vi "Day 2 - part b solution.vi"() -> ()   [LabVIEW 2020]
panel:
  in  "Input":string="A Y\nB X\nB X\nC Y\nB X\nA Z\nB X\nB X\nC Z\nA Z\nC Z\nA X\nA Y\nA Y\nB X\nC Y\nB Z\nA X\nB X\nC Y\nC Y\nA Y\nA Y\nC Y\nB X\nB X\nB X\nA X\nB X\nB X\nC Y\nC Y\nB X\nA Z\nA Z\nB X\nA Z\nC Y\nB X\nB X\nB X\nB X\nB X\nB Z\nA Z\nB X\nA Z\nA X\nB X\nA Z\nB X\nC Y\nA Z\nA Z\nB X\nB X\nB Z\nC Y\nA Y\nB Z\nA Z\nC Z\nB X\nC Y\nC Y\nB Z\nB X\nB X\nB Z\nB X\nB X\nA Y\nA Z\nB Z\nB X\nB Y\nB Z\nB X\nC X\nB Z\nB X\nA Z\nB Z\nB Z\nB X\nA Y\nA Z\nA Y\nB X\nB Z\nB X\nB X\nA Y\nA Y\nB X\nB X\nB X\nC X\nC Y\nB X\nB X\nB Z\nB X\nB X\nB X\nC Y\nB X\nC Y\nA Z\nB X\nB Z\nB X\nC Y\nC Y\nA Z\nA Y\nC Y\nB X\nB X\nB Z\nA Y\nB X\nB X\nB X\nA Y\nB Z\nB X\nA Y\nB Z\nC Y\nA X\nB X\nB X\nA Z\nC Y\nB X\nB Z\nA Y\nA Y\nC Y\nA Y\nC Y\nB X\nB Z\nB X\nC Y\nA Y\nB X\nC Z\nA Z\nC Y\nB X\nB Z\nB X\nB X\nB Z\nB Y\nA Y\nB X\nA Y\nA Z\nA Z\nB X\nC Y\nB Z\nA X\nA Y\nB X\nA Z\nB X\nA Y\nB Y\nB X\nA Y\nB X\nB X\nB X\nB X\nB X\nB X\nB X\nA Z\nB X\nB X\nB Z\nB Z\nB Z\nB Z\nA Y\nB Z\nC Z\nB X\nB X\nB X\nA Z\nB Z\nC Y\nB X\nC Y\nB Z\nB X\nB Z\nB X\nC Z\nA Z\nA Y\nA X\nB X\nB Z\nA Y\nB X\nB X\nB X\nB X\nC Y\nC Y\nA Z\nA Y\nA X\nB X\nB X\nA Y\nB X\nC Y\nA X\nB X\nB X\nB X\nA Z\nC Y\nB Z\nC Y\nA Y\nC Y\nA X\nA Z\nC Z\nA Z\nB X\nB Z\nB X\nB X\nA X\nB X\nB X\nB Z\nA Y\nC Y\nA Z\nC Z\nA Z\nA Z\nA Z\nB Z\nB Z\nB Z\nC Z\nB Y\nC Y\nC Y\nC X\nB X\nC Y\nB X\nB X\nC Y\nB Z\nB X\nC Z\nB X\nA Z\nB Z\nC X\nC Y\nB X\nA Y\nA Z\nB X\nA Z\nA Z\nB X\nB X\nC Z\nB Z\nA Z\nA Z\nC Z\nB X\nA Z\nA X\nB X\nB X\nC Y\nB X\nB Z\nA Z\nB X\nB X\nB X\nB X\nB X\nB X\nB X\nB X\nC Y\nC Y\nB X\nB X\nB X\nC Y\nA X\nB Z\nB X\nB X\nC Z\nB X\nB Z\nB Z\nA Z\nB X\nB Z\nB X\nA Z\nB X\nB X\nB X\nB X\nB X\nC Z\nB X\nB X\nB X\nB Z\nC Y\nC Y\nA Y\nB X\nB Z\nC Y\nB X\nB X\nC Y\nC Y\nB X\nB X\nB X\nB X\nC X\nB Z\nB X\nB Z\nC Y\nA X\nA Z\nB X\nB X\nA Z\nB X\nC Z\nB X\nA Y\nA Z\nB X\nB X\nB X\nB Z\nB X\nA Y\nC Y\nB Z\nB Z\nC Y\nB X\nA Y\nC Y\nB X\nC Z\nB X\nB X\nA Z\nB Z\nB Z\nB X\nA Z\nA Z\nA Y\nB Z\nB X\nB X\nB X\nB X\nB Z\nB X\nB Z\nB X\nA Z\nB X\nB X\nC Z\nC Z\nB X\nC Y\nA Z\nB X\nB Z\nC Z\nC X\nB X\nA Y\nA Y\nB X\nB X\nC Y\nA X\nC Y\nA Y\nA Z\nC Z\nB Z\nA Z\nB X\nB X\nB Z\nC Y\nA Y\nA Y\nB Z\nA Z\nA Z\nB Z\nA Z\nB X\nA Y\nA Y\nC Y\nB X\nB X\nA X\nB X\nC X\nA Y\nA Z\nB X\nB X\nB X\nB X\nB X\nB Z\nB Z\nB Z\nB X\nB X\nA Z\nB X\nC Z\nA Z\nC Y\nB Z\nC Y\nA Y\nC Y\nB X\nB X\nB X\nA Y\nB Z\nB Z\nB X\nB Z\nB X\nB X\nB X\nC Y\nB X\nB Z\nA Z\nB X\nB X\nB X\nC Z\nC Z\nB Z\nB X\nA Z\nA X\nB X\nB X\nB Y\nA Y\nB X\nB X\nC Z\nA Z\nB X\nB Z\nB Z\nA Y\nA Z\nB Z\nB Z\nA Y\nA Y\nA Z\nC Y\nC Y\nB X\nB X\nA Z\nB X\nC Y\nC X\nA Z\nB X\nB X\nB X\nA Y\nC Y\nB Y\nC Y\nC X\nA X\nA Y\nB Z\nB X\nB Z\nA X\nB X\nC Z\nB X\nB X\nA Y\nB Z\nB X\nA Y\nA Y\nB X\nC Y\nB X\nB X\nC Y\nB X\nC Z\nB Z\nB X\nA X\nC Y\nC Y\nB X\nB Z\nB X\nB X\nA Z\nB X\nA Z\nB Z\nB X\nB X\nB Z\nA Y\nC Y\nB Z\nB X\nA Y\nB X\nA X\nC Z\nB X\nB Z\nB Z\nA X\nC Y\nA Z\nB X\nB Z\nA Y\nB X\nC Y\nA Y\nB Z\nC Y\nB X\nB X\nB X\nB X\nB X\nB X\nC Y\nB X\nC Z\nA Y\nC Y\nB X\nC Y\nB Z\nB X\nA X\nB Z\nB X\nC X\nB X\nA Z\nB X\nA Y\nB X\nC Z\nB X\nB Z\nA Y\nB X\nA Z\nA Z\nA Z\nA Y\nA Y\nB X\nA Z\nB X\nB X\nA Y\nA Y\nA Y\nB Z\nC Y\nB Z\nB X\nC Z\nA Y\nC Y\nB X\nB X\nB Z\nB X\nB X\nB X\nC Y\nC Y\nA Y\nB Z\nB Z\nB X\nB X\nB Z\nB X\nA Y\nC Y\nB X\nC X\nB Z\nB X\nB Z\nB Z\nC Y\nB Z\nB X\nC X\nB X\nC Y\nB X\nA Z\nB X\nB X\nB X\nB X\nB X\nC Y\nA Y\nB X\nC Y\nB Z\nB Z\nB X\nC X\nB Z\nC Y\nC X\nC Y\nA Z\nB Z\nC Y\nC X\nB X\nA Y\nC Y\nB X\nC Z\nB Z\nA Y\nC Z\nC X\nB X\nB X\nA Y\nC X\nB X\nB X\nA X\nA Z\nA X\nA Y\nA Y\nC Y\nB X\nC Z\nB X\nC Y\nA Y\nB X\nB X\nB X\nB X\nA Z\nC X\nB X\nB Z\nB X\nB X\nC Y\nB X\nC Z\nB X\nB X\nB X\nB X\nB X\nC Y\nB X\nB X\nA Y\nB X\nC Y\nC Y\nA Y\nB X\nA X\nA Y\nB X\nB Z\nB X\nB Z\nA X\nA Y\nA X\nB X\nC Z\nA Y\nB Z\nA Y\nB Z\nB Z\nB X\nB Z\nB X\nB X\nB X\nB Z\nB X\nB X\nB X\nA Z\nC Z\nC Z\nA X\nA X\nB X\nB X\nA X\nB X\nA X\nA Z\nB Z\nB X\nC Y\nB X\nC Y\nA Y\nC X\nA X\nA Y\nB Z\nB X\nB X\nC Z\nB Y\nA Y\nB Y\nC Y\nA Y\nB X\nB X\nC X\nB Z\nA Y\nB Z\nA Z\nB X\nB X\nA Z\nC Z\nA Y\nB X\nB X\nB Z\nB X\nB X\nB Z\nA X\nA Z\nC Y\nA Y\nA Z\nB X\nC Y\nB Z\nC Y\nB X\nB X\nB Z\nB X\nA Y\nB X\nA Y\nB X\nA Y\nB X\nA Y\nC Y\nA Y\nB Z\nA Y\nB X\nA Z\nC Y\nB X\nB X\nB X\nA X\nB X\nB Z\nA Z\nA Z\nB X\nB Z\nB X\nA Y\nB Z\nB X\nB X\nA Y\nA Y\nC Z\nC Y\nB X\nA X\nA Y\nA X\nC Y\nB X\nC X\nB X\nB X\nA Y\nA Y\nA Y\nB Y\nB X\nB X\nB X\nC Z\nB Z\nC Z\nA X\nB X\nB X\nA Y\nA Z\nB X\nA Y\nB Z\nB Z\nC Y\nB X\nB X\nC X\nB X\nC X\nB X\nB Z\nA X\nB X\nA Z\nA X\nB Z\nA Y\nB X\nB X\nB X\nB X\nB Z\nA Z\nB X\nB Z\nB X\nB Z\nC Y\nB X\nC Y\nB X\nB X\nB X\nA Y\nB X\nA Y\nB X\nB X\nA X\nC Z\nC Y\nA Z\nB X\nA Y\nC Z\nC Y\nC Y\nB Z\nA Y\nB X\nA Y\nB X\nB X\nB Z\nB Z\nB X\nC X\nB Z\nA X\nA Y\nA Y\nB Z\nA Z\nC Y\nB X\nB Z\nA Y\nC Y\nA Y\nA X\nA Z\nB X\nB X\nC Y\nB X\nC Y\nB X\nA X\nB Z\nC X\nB Y\nA Y\nC Y\nB X\nA X\nB X\nB X\nB X\nA Z\nA Y\nB X\nC Z\nB X\nC X\nC Z\nB X\nB X\nC Y\nB X\nB Z\nA Y\nA Y\nB X\nB X\nB Z\nC Y\nB X\nB X\nB X\nA Y\nC Y\nB X\nA Y\nA Z\nC Y\nB X\nA Y\nA Z\nB Z\nA Z\nB X\nC X\nB Z\nA Y\nB Z\nA Y\nC Y\nA X\nA Y\nB X\nC Y\nC Y\nB X\nA X\nB Z\nB X\nB X\nA Z\nA Z\nA Y\nA Y\nB X\nB X\nB X\nA X\nB X\nB X\nB X\nA X\nB Z\nC Z\nA Y\nC Y\nC Y\nC X\nB X\nB Z\nB Z\nB X\nB X\nC Y\nA X\nC Y\nA X\nB X\nB X\nB Z\nB Z\nC Y\nC Y\nA Z\nC Y\nA Z\nB X\nA Z\nA Y\nB Z\nB Z\nB X\nB X\nA Y\nB Z\nB X\nC Z\nA Z\nB Z\nB X\nB Z\nB X\nC Y\nB X\nA Y\nB Z\nC Y\nB Z\nC Z\nB X\nC Z\nB X\nB X\nB X\nC Y\nB X\nB X\nB Z\nA Y\nB X\nB Z\nA Z\nB X\nC Y\nC X\nC Y\nA Z\nB X\nA Z\nB X\nC Z\nA Y\nB Z\nB Z\nA Y\nC Z\nC X\nA Y\nB X\nB Z\nB X\nB X\nB X\nB X\nA X\nB X\nB X\nA Z\nB X\nB X\nA Z\nC Y\nA X\nB Z\nB X\nB X\nA Z\nB X\nA Y\nB Z\nC Y\nB X\nA Y\nC Y\nB Z\nB X\nA Z\nA Z\nB X\nB X\nB Z\nB X\nB X\nA Z\nB X\nB Z\nB Z\nC Y\nA Z\nB X\nA Y\nB X\nB X\nB X\nB Z\nA X\nC Y\nB Z\nB X\nB X\nB X\nB X\nB X\nB Z\nB X\nB Z\nA Z\nB Z\nB X\nC Z\nB Z\nC Z\nA Z\nC X\nA Y\nB Z\nB Z\nB X\nB Z\nB Z\nA Z\nC Z\nA X\nC Y\nC Y\nA Y\nA X\nA Z\nB X\nA Y\nB X\nB X\nC Y\nC Y\nB X\nB Z\nA Y\nB X\nB Z\nB X\nB X\nA Z\nC Y\nB X\nC Y\nA Y\nB Z\nA Z\nA Y\nB X\nA Z\nB Z\nB X\nA Y\nA Y\nA Z\nA X\nB Z\nC Z\nB X\nC Z\nB X\nB Z\nA X\nB X\nB X\nB X\nB X\nC Y\nB X\nA X\nB Z\nA Y\nB X\nA Z\nB X\nB Z\nA Y\nA Y\nA Y\nA Y\nA Z\nC Y\nC Z\nB X\nB Z\nA Y\nB X\nB X\nB X\nA Y\nB Z\nB X\nB Z\nB X\nB X\nB X\nC Y\nC Y\nC X\nB X\nA Y\nA Y\nC Z\nA Y\nA Y\nC X\nA Z\nB X\nB X\nB X\nB X\nC Y\nA Y\nB Z\nA Z\nB X\nC X\nA Z\nB X\nC Y\nB X\nB X\nC Y\nB X\nB X\nB X\nA Y\nB X\nB X\nC Z\nB X\nC Y\nC Y\nB X\nA Z\nB X\nB X\nC Y\nA Y\nB X\nB Z\nB X\nB X\nB X\nC Y\nC Z\nB Z\nC Y\nB X\nB Z\nB X\nB X\nB X\nC Y\nC X\nB X\nA Y\nA Z\nB Z\nA Y\nB X\nB X\nB Y\nC Y\nC X\nB Z\nA Z\nB X\nB X\nA Y\nC Z\nC Y\nB X\nC Y\nA Z\nA Y\nB Z\nB X\nB X\nB X\nB X\nA Z\nA X\nA X\nA X\nC Y\nB Z\nB X\nC Y\nB X\nB X\nA Z\nC Z\nC Z\nB X\nA Y\nB X\nB Z\nB X\nA Y\nA Y\nA Z\nC Y\nA Y\nA Z\nA Y\nA Y\nB X\nA Y\nB X\nA Z\nA Z\nC Y\nB X\nB X\nC Y\nB X\nB X\nB X\nC Y\nA Y\nB X\nA Y\nB Z\nC Y\nB X\nA Y\nB Z\nA Z\nB Z\nA Z\nB X\nC Y\nB X\nB X\nB X\nC Y\nA Y\nB X\nA Y\nC X\nA Z\nB X\nB Y\nB X\nB X\nA Z\nB X\nB X\nB Z\nB X\nC Y\nB X\nB X\nB Z\nB X\nC Y\nB X\nC Y\nB X\nB Z\nA Y\nB X\nB X\nC Z\nB X\nC Y\nA Y\nC Y\nB X\nB Z\nB X\nB X\nB X\nB X\nA Y\nB X\nA Z\nA Y\nA X\nC Y\nB X\nC Y\nB X\nA Z\nC Y\nC Y\nB Z\nB X\nA Y\nB Z\nA Y\nA Y\nB Z\nB Z\nB X\nC Y\nC Y\nB X\nA X\nA Z\nB X\nC Y\nB X\nB X\nB Z\nB X\nB Z\nC Y\nC Z\nC Y\nA Y\nA Z\nB X\nC Y\nA Y\nC X\nB X\nB X\nA Y\nB X\nB X\nB X\nB Z\nB Y\nA X\nA Y\nC Y\nC Y\nA Y\nC Y\nB Z\nB Z\nC Y\nB X\nC Y\nC Z\nA Y\nC X\nA Y\nA Y\nC Y\nC Y\nB X\nA Y\nA X\nB X\nB X\nB Z\nB X\nA Z\nA Y\nA Y\nB X\nB X\nB Z\nB Z\nB X\nB Z\nA Z\nA Y\nA Z\nB X\nC Y\nB Z\nB X\nA Y\nB X\nC X\nB X\nB X\nC Y\nB X\nB X\nB X\nA Y\nA X\nA Y\nB X\nB X\nA Y\nA Y\nA Z\nA Z\nC X\nC Y\nA Z\nC Y\nB Z\nB X\nA Y\nB X\nB Z\nC Z\nA Y\nA Z\nA Y\nB X\nB Z\nB X\nA X\nB Z\nB X\nC Y\nB X\nA Z\nC Z\nA X\nB X\nB X\nA Y\nC Y\nB X\nB X\nB X\nB X\nB X\nA X\nB X\nA Z\nC Z\nB Z\nB X\nC X\nA X\nC Y\nA Y\nA Z\nB X\nA X\nA Z\nA Z\nB X\nB X\nA Z\nC Y\nA Z\nB X\nC Y\nB X\nC Z\nC Y\nC X\nA Z\nC X\nB Z\nB X\nB X\nC Y\nB X\nC Y\nA Z\nA Z\nA Z\nA Y\nA Z\nB X\nB X\nB X\nB Z\nC Y\nC Z\nC Y\nC Y\nC Y\nA Y\nB Z\nA X\nB X\nB X\nB X\nA X\nA Y\nB X\nB Z\nA Z\nA Y\nA Y\nB Z\nB X\nB X\nC Y\nC Y\nC Y\nB X\nC Y\nB X\nB X\nB X\nC Y\nA Y\nA Y\nC Z\nC Y\nB X\nA X\nA Y\nB X\nC Y\nB X\nA Y\nC Y\nA Y\nB X\nB X\nB Z\nA Y\nB Z\nB Z\nB X\nB X\nC X\nC Y\nB X\nB X\nA X\nC Y\nB X\nB Z\nB X\nB X\nA Y\nB X\nB Z\nB Z\nC Y\nB X\nB Z\nB Z\nB Z\nB X\nB X\nA Y\nB X\nB X\nB Z\nC Y\nA Y\nB X\nB Z\nB X\nB X\nA X\nB X\nB X\nB X\nB Z\nB Z\nB Z\nB X\nA Z\nB X\nA Z\nA Y\nB Z\nB X\nA Y\nB X\nB Z\nB X\nA Z\nB X\nB Z\nC Z\nA X\nB X\nB X\nB X\nC Y\nB X\nB X\nA Y\nA Z\nB X\nC Y\nB X\nC Y\nB X\nB Y\nB X\nC Z\nB X\nC Z\nA Y\nB X\nC Z\nB X\nA Y\nC Y\nB X\nB X\nB Z\nC X\nB Z\nB X\nA Z\nB X\nB X\nB X\nB Z\nB X\nA Z\nC Y\nA Y\nB X\nB X\nA Z\nB X\nA Y\nB X\nC Y\nB Z\nB Z\nB X\nB Z\nB X\nB X\nB X\nB X\nB X\nC Y\nA Z\nA Z\nB Z\nA Y\nB Z\nC Y\nA Y\nA Y\nC Y\nA Y\nB Z\nA Y\nA Y\nB X\nB X\nA X\nB X\nC Y\nC Y\nB Z\nB X\nA Z\nB Z\nB X\nA Z\nB Z\nA Y\nA Y\nA Y\nA Y\nA Z\nA Y\nB X\nB Z\nA Y\nB X\nA Z\nB Z\nC X\nB X\nB X\nB Z\nB Z\nB X\nB X\nB X\nB X\nB X\nB X\nB X\nB Z\nB X\nB X\nB X\nB X\nB X\nB Z\nB X\nB X\nB Z\nB Z\nB X\nA Y\nB Z\nB X\nA Z\nA Y\nA Z\nB X\nB X\nA X\nB Y\nA Z\nB X\nC Z\nA Z\nB X\nB Z\nB X\nB X\nB X\nA Y\nC Y\nB X\nB X\nB X\nA Y\nB X\nA Z\nB X\nB X\nB X\nB Z\nB Z\nC X\nC Y\nB X\nB X\nC Y\nB X\nB X\nB X\nA X\nA Z\nA Z\nB Z\nB Z\nB X\nA Y\nB X\nC Y\nB Z\nC Y\nC Z\nA Y\nA Y\nB X\nB X\nA Z\nB X\nB X\nB Z\nB X\nB X\nA Z\nB X\nB X\nB X\nC Y\nB X\nB X\nC Y\nB X\nB X\nB Z\nB X\nB X\nA Y\nC Y\nA X\nC Y\nB X\nB X\nA Z\nA Y\nB X\nA X\nB Z\nA Y\nB X\nB X\nA Y\nB X\nC X\nB X\nB X\nB Z\nB Z\nB X\nB Z\nB X\nB X\nA Y\nA Y\nB X\nB Z\nC Y\nB X\nB X\nB X\nA Z\nB X\nA Y\nB X\nC Y\nA X\nA Y\nB X\nB X\nC Y\nB X\nB X\nB X\nA Z\nB Z\nB X\nC X\nA Z\nC Y\nB X\nB Z\nB X\nB X\nA Z\nB X\nA Y\nC Y\nB X\nB Z\nC X\nA Z\nA Z\nB Z\nB Z\nA X\nB X\nA Y\nB X\nB X\nB X\nB X\nA Z\nB Z\nB Z\nC Y\nA X\nA Y\nA Y\nA Z\nB X\nA Y\nB Z\nC Y\nB Z\nB X\nA Z\nB Z\nB X\nB Z\nB Z\nB Z\nB X\nC Y\nB X\nB X\nA Y\nB X\nC X\nA Y\nA Z\nA Y\nB X\nC Y\nB Z\nB X\nB X\nA X\nB X\nB X\nA Y\nA Z\nC Z\nA Y\nB X\nB X\nC Y\nA X\nA Z\nB X\nB Z\nB Z\nC Y\nA Z\nC Y\nA Z\nC Y\nC Y\nB Z\nC Y\nB X\nC Y\nC Y\nB X\nB Z\nC X\nC Y\nA Y\nB X\nC Y\nB X\nB X\nC Y\nB Z\nB Z\nA Z\nA Z\nC Y\nB X\nB Z\nB X\nB X\nB X\nC Y\nB X\nC Y\nA Z\nA Z\nB X\nB X\nA Y\nA X\nB X\nA Z\nA Y\nC Y\nB X\nA Y\nA Y\nB X\nA X\nA Z\nA Y\nA Z\nC Y\nC Y\nC Y\nA Y\nB X\nB X\nA Y\nC Y\nB X\nA X\nC Y\nC Y\nA Y\nC Y\nC Y\nB Z\nC Y\nB X\nC Y\nB X\nB X\nB X\nA Y\nB Y\nB X\nC X\nB X\nA X\nA Y\nC Y\nC Y\nB X\nB X\nA Y\nB X\nB X\nA Y\nC Y\nC X\nA Y\nB X\nB Z\nB Z\nB Z\nB X\nA Z\nB X\nB X\nA Y\nB X\nB X\nA Y\nB Z\nA Y\nB X\nB X\nB Z\nA Z\nA Y\nA Z\nA Y\nC Y\nB X\nC X\nB X\nB X\nA Z\nB X\nB Z\nB X\nA Z\nC Y\nB X\nB X\nB Z\nA Z\nA Y\nB X\nB Y\nA Y\nA Z\nA Y\nC Z\nB X\nB X\nB X\nA Z\nB X\nB X\nB X\nA Y\nB Z\nC Y\nC Y\nA Z\nA Z\nA Y\nB X\nA Y\nB Z\nC Y\nB X\nB Z\nA Y\nB X\nA Y\nC Y\nB X\nB X\nA Y\nA Z\nA Z\nA Z\nB X\nB X\nA Z\nB X\nB X\nB Z\nA X\nB Z\nA Z\nB X\nC Y\nC X\nA Z\nB X\nA Y\nB Y\nB Z\nB X\nB X\nA Y\nB X\nA Z\nA Z\nC X\nB X\nB Z\nA Y\nC Y\nA Y\nB X\nB Z\nB X\nA Z\nB Z\nC Y\nB Z\nB X\nB X\nB X\nA Y\nB X\nB X\nA Z\nC Y\nB X\nC Y\nB X\nC Y\nA Z\nA Y\nA X\nC Y\nB X\nB X\nB Z\nB X\nA Y\nA Y\nB X\nB X\nA Z\nC Y\nB Z\nB X\nB X\nA X\nA Y\nB Z\nC Y\nA Z\nC Y\nA Z\nB X\nA Y\nB X\nA Y\nB X\nB X\nC X\nB Y\nC Z\nA Z\nC Y\nB X\nB X\nB Z\nC Z\nA X\nA Y\nA Z\nB X\nC Y\nB Z\nB Z\nA Y\nB X\nB X\nA Y\nA Z\nB X\nB X\nA Z\nB X\nB X\nB Z\nA X\nB X\nA X\nA Y\nC Y\nB X\nB Z\nA Y\nB X\nA X\nB X\nB X\nB Z\nB X\nB X\nA Y\nB X\nB X\nA Y\nA Y\nC Y\nB Z\nB X\nA X\nA Z\nB X\nB X\nC Z\nB X\nB X\nB X\nB X\nB X\nC Y\nC Y\nC X\nB X\nB X\nB Z\nB Z\nB X\nA Y\nB Z\nB Z\nB Z\nB X\nB X\nB X\nB X\nA Y\nA Y\nB X\nC Y\nC Y\nB X\nB X\nA Y\nC Y\nA Z\nC Y\nB X\nC Z\nB X\nB Z\nB X\nC Y\nC Y\nB X\nB X\nB X\nC Y\nB X\nB X\nA X\nB X\nC Y\nA Y\nB X\nB X\nB X\nC X\nC Y\nA Y\nB X\nB X\nC Y\nA Y\nB X\nA Y\nA Y\nB Z\nC Y\nB Z\nA Y\nA Z\nC Y\nB X\nC Y\nB X\nC Y\nC Y\nB X\nB X\nB X\nB Z\nA Y\nB X\nB X\nB X\nA Y\nB X\nB X\nA Y\nB X\nA Y\nC Y\nA Z\nB X\nB X\nC Y\nB X\nB X\nA Y\nA Z\nC Y\nB X\nB Z\nB Z\nB X\nC Y\nB X\nA Y\nC X\nC Y\nB X\nB X\nB Z\nC Y\nB X\nB X\nC Y\nC Y\nB X\nC Y\nB Z\nC Y\nC X\nB Z\nC Y\nB Z\nC Y\nA X\nB Z\nB Z\nB X\nB X\nC Y\nB X\nC Y\nB X\nB X\nB X\nA Y\nB X\nC Y\nB Z\nC Y\nC Y\nA Y\nC Z\nA Y\nB X\nA Z\nC Z\nC Y\nB X\nB X\nA Y\nB Z\nB X\nC Y\nB X\nB Z\nA Z\nB Z\nA Y\nC Y\nA Z\nB X\nB X\nC Y\nC Y\nB X\nB X"
  out "Score":i32
  # "Advent of code 2022 day 2 pt b"
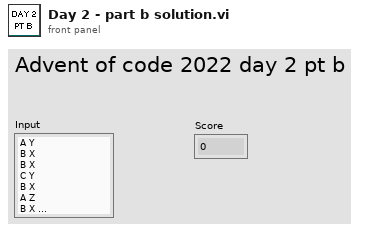
[diagram p1: front panel]
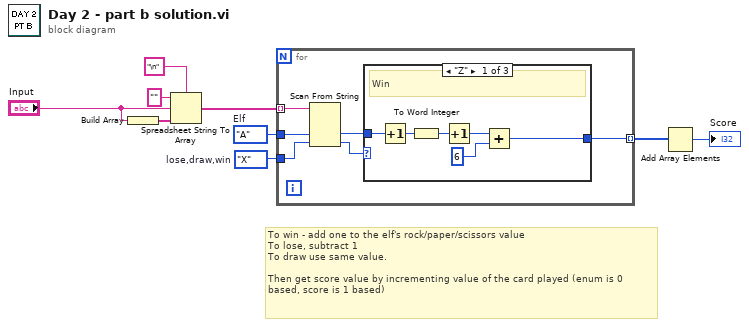
[diagram p0: block diagram]
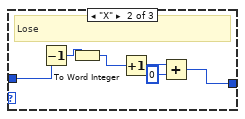
[diagram p2: hidden frame]
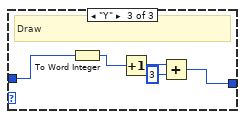
[diagram p3: hidden frame]
diagram:
  w2 = enum16{"X", "Y", "Z"}."X"  # lose,draw,win
  w1 = enum16{"A", "B", "C"}."A"  # Elf
  # "To win - add one to the elf's rock/paper/scissors value\nTo lose, subtract 1\nTo draw use same value.\n\nThen get score value by incrementing value of the card played (enum is 0 \nbased, score is 1 based)"
  n1 = Build Array("Input") -> (w9:string[])
  n2 = Spreadsheet String To Array(delimiter (Tab)="\n", format string="", spreadsheet string="Input", array type (2D Dbl)=w9) -> (array=w6:string[])
  n3 = for {
    tunnel: w6 -> [w15] mode=indexing
    tunnel: [w12] -> w3 mode=indexing
    tunnel: w2 -> [w11]
    tunnel: w1 -> [w10]
    n4 = Scan From String(input string=w15, default 1=w10, default 2=w11) -> (output 1=w13:enum16{"A", "B", "C"}, output 2=w14:enum16{"X", "Y", "Z"})  [unwired: 3 in, 3 out]
    n5 = case shown="\"Z\"" w14 {
      tunnel: w13 -> [w21 w27 w28]
      tunnel: [w16 w22 w29] -> w12
      frame "Z" {
        # "Win"
        n6 = Increment(x=w21) -> (x+1=w20:enum16{"A", "B", "C"})
        n7 = To Word Integer(number=w20) -> (16bit integer=w19:i16)
        n8 = Increment(x=w19) -> (x+1=w18:i16)
        n9 = Add(x=w18, y=i16 6) -> (x+y=w16:i16)
      }
      frame "X" {
        # "Lose"
        n10 = Decrement(x=w27) -> (x-1=w26:enum16{"A", "B", "C"})
        n11 = To Word Integer(number=w26) -> (16bit integer=w25:i16)
        n12 = Increment(x=w25) -> (x+1=w24:i16)
        n13 = Add(x=w24, y=i16 0) -> (x+y=w22:i16)
      }
      frame "Y" {
        # "Draw"
        n14 = To Word Integer(number=w28) -> (16bit integer=w32:i16)
        n15 = Increment(x=w32) -> (x+1=w31:i16)
        n16 = Add(x=w31, y=i16 3) -> (x+y=w29:i16)
      }
    }
  }
  n17 = Add Array Elements(numeric array=w3) -> (sum=→"Score":i16)
